vi "TestInitializeTriggeredSubscription_RejectOldValue.vi"(8 "error in (no error)":errorcluster, 11 "TestCase in":refnum<class "TestSubscriptionPolicy.lvclass">) -> (0 "error out":errorcluster, 3 "TestCase out":refnum<class "TestSubscriptionPolicy.lvclass">)   [LabVIEW 2017, in "TestSubscriptionPolicy.lvclass"]
uses:
  TestSubscriptionPolicy.lvclass
  TriggeredSubscription/Trigger Condition.ctl
  TriggeredSubscription/TriggeredSubscription.lvclass/TriggeredSubscription.ctl
  Transport/QueueTransport/QueueTransport.lvclass/QueueTransport.ctl
  IMediator/ISubscriptionPolicy/ISubscriptionPolicy.lvclass/ISubscriptionPolicy.ctl
  Transport/QueueTransport/QueueTransport.lvclass
  C:/Git/mva-framework/Framework/IMediator/ITransport/ITransport.lvclass
  TriggeredSubscription/TriggeredSubscription.lvclass
  C:/Git/mva-framework/Framework/IMediator/ISubscriptionPolicy/ISubscriptionPolicy.lvclass
  <vilib>/Utility/error.llb/Error Cluster From Error Code.vi
  IMediator/ISubscriptionPolicy/ISubscriptionPolicy.lvclass
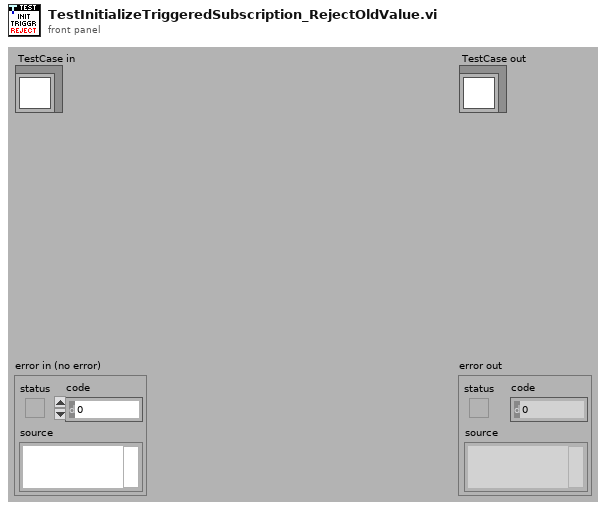
[diagram p1: front panel]
types:
  T1 = typedef "SubscriptionPolicy.lvlib/TriggeredSubscription.lvclass/Trigger Condition.ctl" = enum16{"Equal", "Not equal", "Greater than", "Less than", "Greater or equal", "Less or equal"}
  T2 = typedef "IMediator.lvlib/ISubscriptionPolicy.lvclass/ISubscriptionPolicy Reference.ctl" = refnum<data-value>
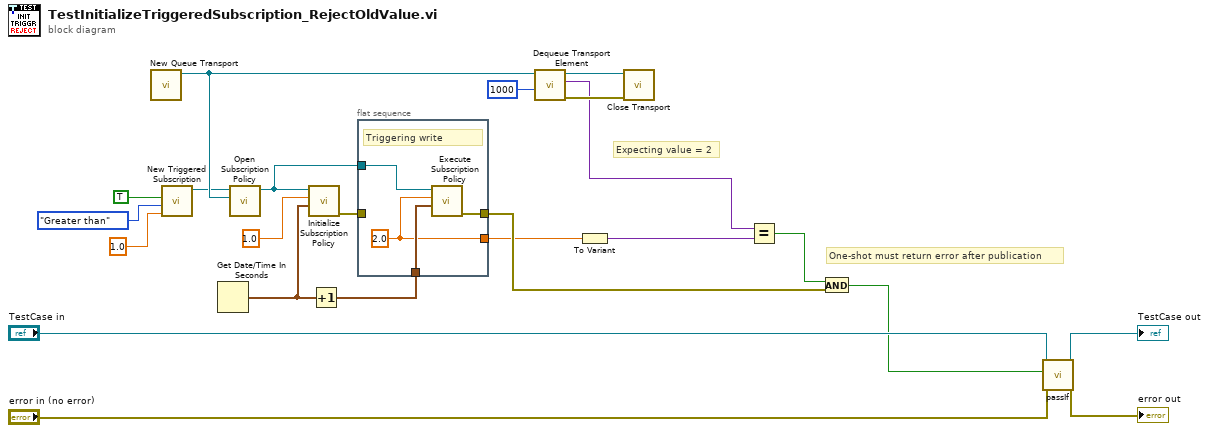
[diagram p0: block diagram]
diagram:
  # "One-shot must return error after publication"
  # "Expecting value = 2"
  n1 = call "New Queue Transport.vi"() -> ("QueueTransport"=w19:refnum<class "QueueTransport.lvclass">)  [unwired: 10 in, 1 out]
  n2 = call "New Triggered Subscription.vi"("Trigger Value"=1.0, "Trigger Condition"=Trigger_Condition."Greater than", "Ignore Past Updates? (F)"=TRUE) -> ("TriggeredSubscription Out"=w15:refnum<class "TriggeredSubscription.lvclass">)  [unwired: 8 in]
  n3 = Get Date/Time In Seconds() -> (seconds since 1Jan1904=w6:timestamp)
  n4 = call "Open Subscription Policy.vi"("Transport"=w19, "SubscriptionPolicy"=w15) -> ("Subscription Policy"=w7:T2)  [unwired: 8 in, 1 out]
  n5 = call "Initialize Subscription Policy.vi"("Last Publish Time"=w6, "Last Topic Value"=1.0, "Subscription Policy"=w7) -> ("Error Out (Do Not Subscribe?)"=w2:errorcluster)  [unwired: 8 in]
  n6 = Increment(x=w6) -> (x+1=w5:timestamp)
  n7 = flat-sequence {
    tunnel: w7 -> [w27]
    tunnel: w5 -> [w26]
    tunnel: [w25] -> w4
    tunnel: [w24] -> w3
    tunnel: w2 -> [_]
    frame #0 {
      w24 = 2.0
      # "Triggering write"
      n8 = call "Execute Subscription Policy.vi"("Publish Time"=w26, "New Topic Value"=w24, "Subscription Policy"=w27) -> ("error out (Unsubscribe?)"=w25:errorcluster)  [unwired: 8 in]
    }
  }
  n9 = call "Dequeue Transport Element.vi"("Timeout In ms (-1)"=1000, "QueueTransport in"=w19) -> ("error out"=w16:errorcluster, "Data"=w1:variant, "QueueTransport out"=w17:refnum<class "QueueTransport.lvclass">)  [unwired: 6 in, 1 out]
  n10 = To Variant(anything=w3) -> (Variant=w12:variant)
  n11 = call-dynamic "Close Transport.vi"("error in (no error)"=w16, "QueueTransport in"=w17) -> ()  [unwired: 9 in, 1 out]
  n12 = Equal?(x=w1, y=w12) -> (x = y?=w11:bool)
  n13 = And(x=w11, y=w4) -> (x .and. y?=w10:bool)
  n14 = call-dynamic "passIf.vi"("error in (no error)"="error in (no error)", "pass"=w10, "TestCase in"="TestCase in") -> ("error out"=→"error out":errorcluster, "TestCase out"=→"TestCase out":refnum<class "TestSubscriptionPolicy.lvclass">)  [unwired: 7 in]
